vi "BBB Expand File System.vi"(8 "Error In":errorcluster, 11 "Install LV Data":T1={"SSH Session"=refnum, "Status Log"="", "Detailed Log"="", "Credentials"={"Hostname or IP"="192.168.7.2", "Username"="root", "Password"=""}, "Target Info"={"OS Version"="", "CPU"="", "Systemd Version"="", "Internet Access"=FALSE, "Device Type"="", "LV Installed Ver"="", "LV Available Ver"="", "LV Upgrade Available"=FALSE, "Hostname"="", "NIC Info"=[]}, "Reboot Required?"=FALSE}) -> (0 "Error Out":errorcluster, 2 "Fixed?":bool, 3 "Install LV Data":T1={"SSH Session"=refnum, "Status Log"="", "Detailed Log"="", "Credentials"={"Hostname or IP"="192.168.7.2", "Username"="root", "Password"=""}, "Target Info"={"OS Version"="", "CPU"="", "Systemd Version"="", "Internet Access"=FALSE, "Device Type"="", "LV Installed Ver"="", "LV Available Ver"="", "LV Upgrade Available"=FALSE, "Hostname"="", "NIC Info"=[]}, "Reboot Required?"=FALSE})   [LabVIEW 2014, in "LMH-LINX.lvlib"]
uses:
  <vilib>/MakerHub/LINX/LMH-LINX.lvlib
  <vilib>/MakerHub/LINX/Private/Utilties/Target Management/Install LV Data.ctl
  C:/Program Files (x86)/National Instruments/LabVIEW 2014/vi.lib/MakerHub/LINX/Resources/Renci.SshNet.dll
  Resources/Renci.SshNet.dll
  <vilib>/MakerHub/LINX/Private/Utilties/Target Management/Target Info.ctl
  <vilib>/MakerHub/LINX/Private/Utilties/Target Management/NIC Info.ctl
  <vilib>/MakerHub/LINX/Private/Utilties/Target Management/NIC Mode.ctl
  <vilib>/MakerHub/LINX/Private/Utilties/Target Management/Status FGV States.ctl
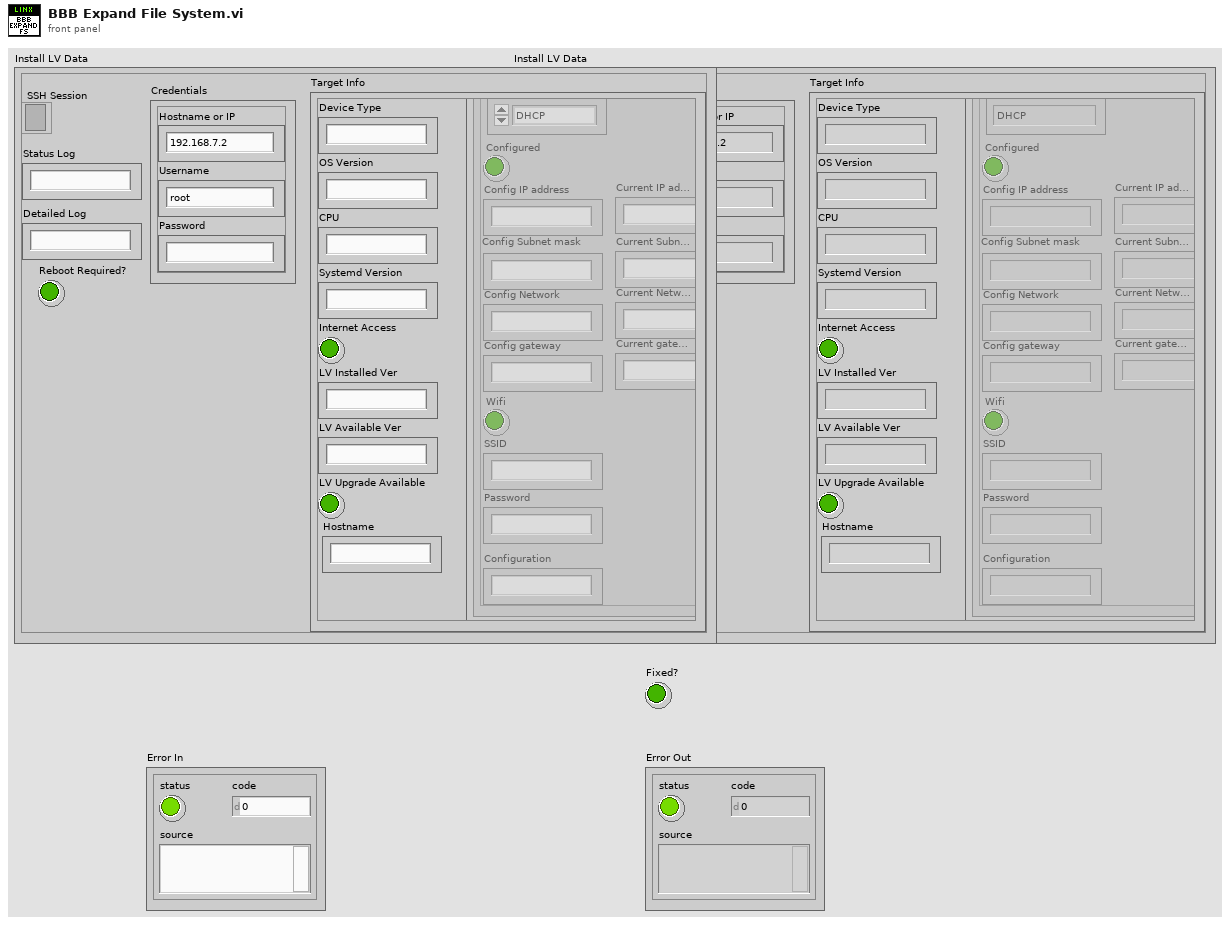
[diagram p1: front panel]
types:
  T1 = typedef "LMH-LINX.lvlib/Install LV Data.ctl" = cluster{"SSH Session":refnum<k24>, "Status Log":string, "Detailed Log":string, "Credentials":cluster{"Hostname or IP":string, "Username":string, "Password":string}, "Target Info":T2, "Reboot Required?":bool}
  T2 = typedef "LMH-LINX.lvlib/Target Info.ctl" = cluster{"OS Version":string, "CPU":string, "Systemd Version":string, "Internet Access":bool, "Device Type":string, "LV Installed Ver":string, "LV Available Ver":string, "LV Upgrade Available":bool, "Hostname":string, "NIC Info":T3[]}
  T3 = typedef "LMH-LINX.lvlib/NIC Info.ctl" = cluster{"Name":string, "NIC Mode":T4, "Configured":bool, "Config IP address":string, "Config Subnet mask":string, "Config Network":string, "Config gateway":string, "Wifi":bool, "SSID":string, "Password":string, "Configuration":string, "Current IP address":string, "Current Subnet mask":string, "Current gateway":string, "Current Network":string}
  T4 = typedef "LMH-LINX.lvlib/NIC Mode.ctl" = enum16{"DHCP", "Static", "Loopback"}
  T5 = typedef "LMH-LINX.lvlib/Status FGV States.ctl" = enum16{"Init", "Append", "Append History Only", "Set", "Get"}
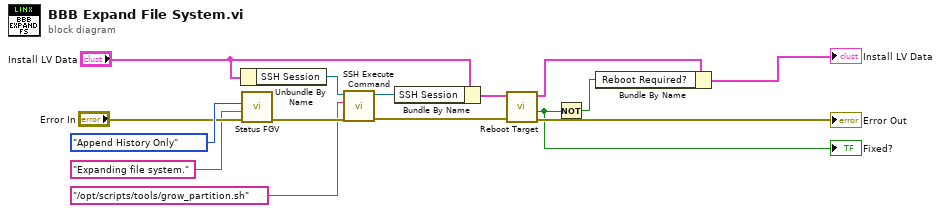
[diagram p0: block diagram]
diagram:
  n1 = Unbundle By Name("Install LV Data") -> ("SSH Session"=w6:refnum<k24>)
  n2 = call <vilib>:"Status FGV.vi"("Error In"="Error In", "Status"="Expanding file system.", "Status FGV State"=Status_FGV_States."Append History Only") -> ("Error Out"=w8:errorcluster)  [unwired: 6 in, 2 out]
  n3 = call <vilib>:"SSH Execute Command.vi"("Error In"=w8, "Command"="/opt/scripts/tools/grow_partition.sh", "SSH Session"=w6) -> ("Error Out"=w7:errorcluster, "SSH Session"=w5:refnum<k24>)  [unwired: 6 in, 1 out]
  n4 = Bundle By Name(cluster="Install LV Data", "SSH Session"=w5) -> (w3:T1)
  n5 = call <vilib>:"Reboot Target.vi"("Error In"=w7, "Install LV Data"=w3) -> ("Error Out"=→"Error Out":errorcluster, "Connected?"=w1:bool, "Install LV Data"=w12:T1)  [unwired: 7 in]
  "Fixed?" <- w1
  n6 = Not(x=w1) -> (.not. x?=w10:bool)
  n7 = Bundle By Name(cluster=w12, "Reboot Required?"=w10) -> (→"Install LV Data":T1)
